vi "Test Get All.vi"() -> ()   [LabVIEW 2019, in "instrument.Cryostation.lvclass"]
uses:
  instrument.Cryostation.lvclass
  C:/Program Files (x86)/National Instruments/LabVIEW 2019/user.lib/LevyLab/Levylab Instruments/SMOs/Instrument/Instrument.lvclass
  <userlib>/LevyLab/Levylab Instruments/SMOs/Instrument/Instrument.lvclass/Instrument.ctl
  <userlib>/LevyLab/Levylab Instruments/SMOs/Instrument/Instrument.lvclass
panel:
  out "getAll":variant=variant(cluster{"Chamber Pressure (mTorr)":dbl, "Compressor Return Pressure (MPa)":dbl, "Compressor Supply Pressure (MPa)":dbl, "Compressor Speed (Hz)":dbl, "Cold Head Speed (Hz)":dbl, "Platform Heater Power (W)":dbl, "Platform Stability (K)":dbl, "Platform Temperature (K)":dbl, "Stage 1 Heater Power (W)":dbl, "Stage 1 Temperature (K)":dbl, "Stage 2 Heater Power (W)":dbl, "Stage 2 Temperature (K)":dbl, "Sample Stability (K)":dbl, "Sample Temperature (K)":dbl, "Temperature Set Point (K)":dbl, "User Stability (K)":dbl, "User Temperature (K)":dbl, "User Temperature Set Point (K)":dbl, "Alarm State":string, "Compressor Run State":string, "Case Valve State":string, "Idle State":string, "Nitrogen State":string, "Vent Valve State":string} {"Chamber Pressure (mTorr)"=769917.3, "Compressor Return Pressure (MPa)"=1.692, "Compressor Supply Pressure (MPa)"=1.68, "Compressor Speed (Hz)"=14.0, "Cold Head Speed (Hz)"=70.0, "Platform Heater Power (W)"=0.0, "Platform Stability (K)"=0.00253, "Platform Temperature (K)"=294.105, "Stage 1 Heater Power (W)"=0.0, "Stage 1 Temperature (K)"=292.75, "Stage 2 Heater Power (W)"=0.0, "Stage 2 Temperature (K)"=292.8, "Sample Stability (K)"=0.00238, "Sample Temperature (K)"=294.172, "Temperature Set Point (K)"=5.0, "User Stability (K)"=-0.1, "User Temperature (K)"=-0.1, "User Temperature Set Point (K)"=-0.1, "Alarm State"="F", "Compressor Run State"="Off", "Case Valve State"="Closed", "Idle State"="T", "Nitrogen State"="T", "Vent Valve State"="Closed"})
  in  "address":string="130.49.180.92"
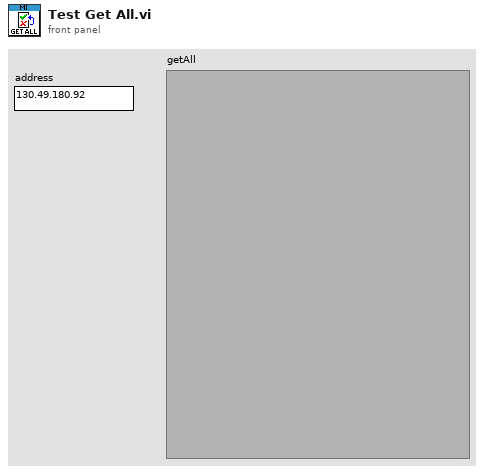
[diagram p1: front panel]
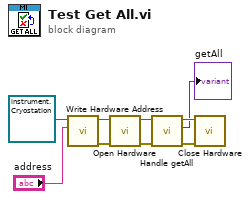
[diagram p0: block diagram]
diagram:
  n1 = call <userlib>:"Write Hardware Address.vi"("Address"="address", "Instrument in"=refnum<class "instrument.Cryostation.lvclass"> refnum ("instrument.Cryostation in")) -> ("error out"=w4:errorcluster, "Instrument out"=w8:refnum<class "instrument.Cryostation.lvclass">)  [unwired: 8 in]
  n2 = call-dynamic "Open Hardware.vi"("error in (no error)"=w4, "instrument.Cryostation in"=w8) -> ("error out"=w3:errorcluster, "instrument.Cryostation out"=w7:refnum<class "instrument.Cryostation.lvclass">)  [unwired: 8 in]
  n3 = call-dynamic "Handle getAll.vi"("error in (no error)"=w3, "instrument.Cryostation in"=w7) -> ("error out"=w2:errorcluster, "getAll"=→"getAll":variant, "instrument.Cryostation out"=w6:refnum<class "instrument.Cryostation.lvclass">)  [unwired: 7 in]
  n4 = call-dynamic "Close Hardware.vi"("error in (no error)"=w2, "instrument.Cryostation in"=w6) -> ()  [unwired: 8 in, 2 out]
